vi "DSWrite Indices (DNet CommandRegister Buffer).vi"(8 "error in":errorcluster[](array[cluster]), 9 "Indices":i32[](array[numeric]), 10 "data":bool[](array[boolean]), 11 "connection in":refnum<k13>[](array[refnum])) -> (0 "error out":errorcluster[](array[cluster]), 3 "connection out":refnum<k13>[](array[refnum]))   [LabVIEW 2011]
panel:
  in  "ms timeout (10000)":i32
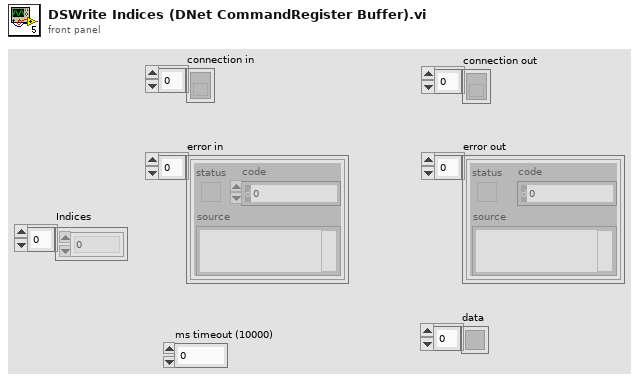
[diagram p1: front panel]
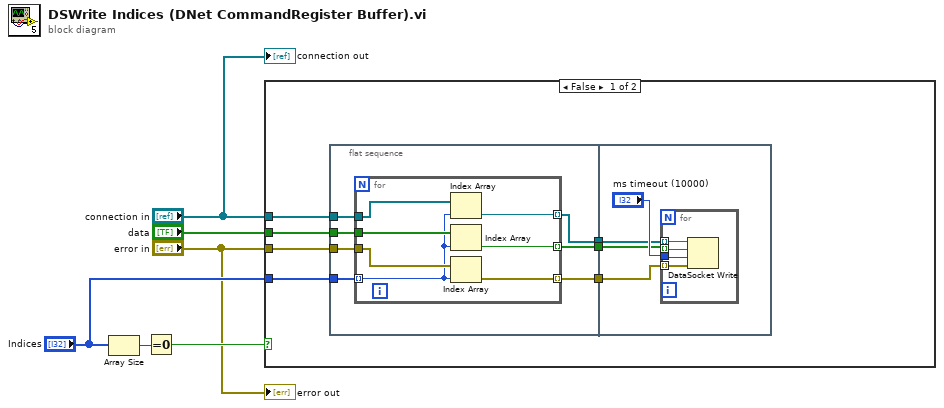
[diagram p0: block diagram]
diagram:
  n1 = Array Size(array="Indices") -> (size(s)=w5:i32)
  n2 = Equal To 0?(x=w5) -> (x = 0?=w6:bool)
  n3 = case shown="False" w6 {
    tunnel: "Indices" -> [w13 _]
    tunnel: "connection in" -> [w7 _]
    tunnel: "data" -> [w12 _]
    tunnel: "error in" -> [w8 _]
    frame False {
      n4 = flat-sequence {
        tunnel: w13 -> [w18]
        tunnel: w7 -> [w20]
        tunnel: w12 -> [w19]
        tunnel: w8 -> [w17]
        tunnel: [w14] -> w11
        tunnel: [w16] -> w10
        tunnel: [w15] -> w9
        tunnel: w11 -> [w30]
        tunnel: w10 -> [w29]
        tunnel: w9 -> [w28]
        frame #0 {
          n5 = for {
            tunnel: w20 -> [w27]
            tunnel: w19 -> [w26]
            tunnel: w18 -> [w24] mode=indexing
            tunnel: w17 -> [w25]
            tunnel: [w23] -> w15 mode=indexing
            tunnel: [w22] -> w16 mode=indexing
            tunnel: [w21] -> w14 mode=indexing
            n6 = Index Array(array=w27, index=w24) -> (element=w21:refnum<k13>)
            n7 = Index Array(array=w26, index=w24) -> (element=w22:bool)
            n8 = Index Array(array=w25, index=w24) -> (element=w23:errorcluster)
          }
        }
        frame #1 {
          n9 = for {
            tunnel: w30 -> [w35] mode=indexing
            tunnel: w28 -> [w34] mode=indexing
            tunnel: "ms timeout (10000)" -> [w33]
            tunnel: w29 -> [w32] mode=indexing
            n10 = DataSocket Write(8:w34, 9:w33, 10:w32, 11:w35) -> ()  [unwired: 3 out]
          }
        }
      }
    }
    frame True {
    }
  }
  "connection out" <- "connection in"
  "error out" <- "error in"
